vi "AlliGator Draw Phasor Plot SEPL v2.vi"(7 "Font, Size & Style":T1, 8 "Error In":errorcluster, 9 "Overlay Group":string="SEPL", 10 "Phasor Plot Reference Points":T2, 11 "Phasor Plot Image  in":T3) -> (0 "Error Out":errorcluster, 3 "Phasor Plot Image out":T3)   [LabVIEW 2021, in "AlliGator Phasor Plot.lvlib"]
doc: "Draws the selected SEPL on the Phasor Plot image."
uses:
  AlliGator Phasor Plot.lvlib
  <vilib>/vision/Image Controls.llb/IMAQ Image.ctl
  Phasor Ratio/AlliGator Phasor Plot Reference Points.ctl
  Settings/AlliGator Phasor Plot Graphics Options.ctl
  Settings/AlliGator Settings List.ctl
  92607714-a441-4b97-ba68-5943c871a3f7.vi
  Phasor Graph/AlliGator Phasor Graph.lvlib
  Settings/AlliGator Settings.lvlib
  Phasor Ratio/AlliGator Phasor Ratio.lvlib
panel:
  # "see the AlliGator License on the block diagram (Ctrl+E or Window:Show Block Diagram)"
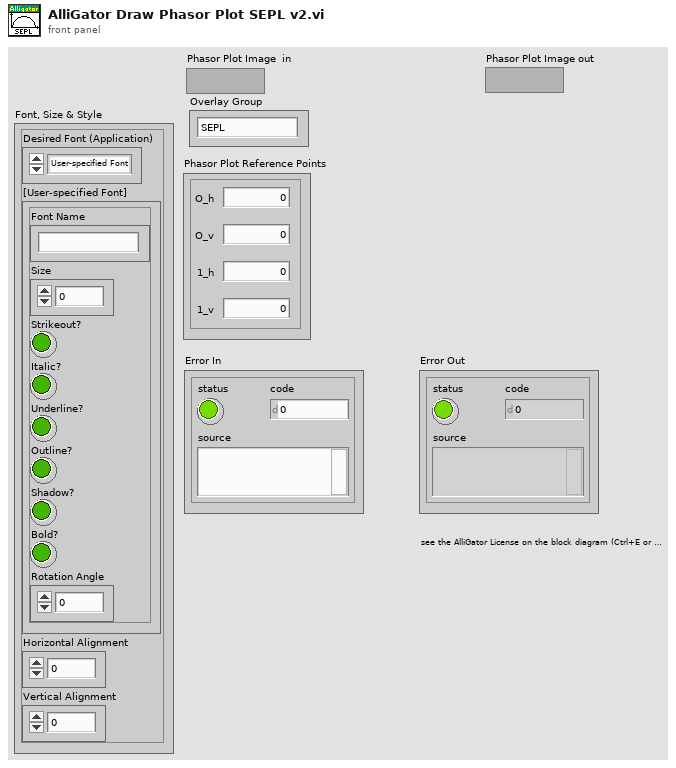
[diagram p1: front panel]
types:
  T1 = cluster{"Desired Font (Application)":enum16{"User-specified Font", "Application Font", "System Font", "Dialog Font"}, "[User-specified Font]":cluster{"Font Name":string, "Size":i16, "Strikeout?":bool, "Italic?":bool, "Underline?":bool, "Outline?":bool, "Shadow?":bool, "Bold?":bool, "Rotation Angle":dbl}, "Horizontal Alignment":i16, "Vertical Alignment":i16}
  T2 = typedef "AlliGator Phasor Ratio.lvlib/AlliGator Phasor Plot Reference Points.ctl" = cluster{"O_h":dbl, "O_v":dbl, "1_h":dbl, "1_v":dbl}
  T3 = typedef "IMAQ Image.ctl" = refnum<image>
  T4 = typedef "AlliGator Settings.lvlib/AlliGator Phasor Plot Graphics Options.ctl" = cluster{"UC Color":u32, "Show UC Tau Ticks":bool, "SEPL Color":u32, "Show SEPL Tau Ticks":bool, "Axes Color":u32, "Show (g,s) Ticks":bool, "Show UC":bool, "Show SEPL":bool, "Show Axes":bool, "Show UC Tau Labels":bool, "Show SEPL Tau Labels":bool, "Show (g,s) Labels":bool, "UC Label Size":i16, "UC Label Distance":dbl, "SEPL Label Size":i16, "SEPL Label Distance":dbl, "Axes Label Size":i16, "Axes Label Distance":dbl}
  T5 = typedef "AlliGator Settings.lvlib/AlliGator Settings List.ctl" = enum16{"GUI:Visible Settings Tab", "GUI:Last Run Version", "Source Image:Use Image Histogram for Contrast", "Source Image:Low Count Pixels Rejection Options", "Source Image:High Count Pixels Rejection Options", "Source Image:Use Image Brightness", "Source Image:Blend Overlay with Image Background", "Source Image:Use Fixed ROI Diameter", "Source Image:ROI Diameter", "Source Image:ROI Center Color", "Source Image:Peak Threshold", "Source Image:Intensity Threshold", "Source Image:Image Binning Options", "Source Image:Image Smoothing Options", "Source Image:Image Histogram Active", "Source Image:Invert Binary Mask", "Source Image:Hot Pixel Removal", "Source Image:Overlay Analyzed ROI Center", "Source Image:Auto-Adjust Contrast", "Source Image:Histogram Lower Percentile", "Source Image:Histogram Upper Percentile", "Source Image:Save Source Image", "Source Image:Scale Bar Options", "Source Image:Image Resolution (Pixel Size)", "Source Image:Flatfield Correction", "Source Image:Show Dead Left Columns Correction", "Source Image:Dead Left Columns Correction", "Source Image:Image Pre-Processing Operations Order", "Source Image:Overlay ROI Median", "Source Image:Median Overlay Color", "Data Information:Gate Width", "Data Information:Nanotime Gate Separation", "Data Information:Macrotime Gate Separation", "Data Information:Gate Step", "Data Information:# Gates", "Data Information:Gate Image Exposure", "Data Information:Gate Image Integration", "Data Information:Gates to Skip", "Data Information:Gates to Keep", "Data Information:Define Gates to", "Data Information:Channel Name", "Data Information:Available Channel Names", "Data Information:Channel Arithmetic", "Data Information:Background File Subtraction", "Data Information:Background File", "Data Information:Background Scaling Factor", "Data Information:Background Pile-up Correction", "Data Information:Background Pixel Well Capacity", "Data Information:Laser Period", "Data Information:SYNC Period", "Data Information:Pile-up Correction", "Data Information:Pixel Well Capacity", "Data Information:Dataset Scaling Factor", "Fluorescence Decay_Decay Pre-Processing:Reverse Gates", "Fluorescence Decay_Decay Pre-Processing:Verbose Decay Pre-Processing", "Fluorescence Decay_Decay Pre-Processing:Use Decay Pre-Processing", "Fluorescence Decay_Decay Pre-Processing:Background Subtraction", "Fluorescence Decay_Decay Pre-Processing:Background Definition Range", "Fluorescence Decay_Decay Pre-Processing:Baseline Subtraction Method", "Fluorescence Decay_Decay Pre-Processing:Decay Pre-Processing Operations Order", "Fluorescence Decay_Decay Pre-Processing:Smoothing Parameter", "Fluorescence Decay_Decay Pre-Processing:Shift Decay", "Fluorescence Decay_Decay Pre-Processing:Decay Shift Parameters", "Fluorescence Decay_Decay Pre-Processing:Fold Decay", "Fluorescence Decay_Decay Pre-Processing:# Folds", "Fluorescence Decay_Decay Pre-Processing:1-Normalize Decay", "Fluorescence Decay_Decay Pre-Processing:[0-1]-Normalize Decay", "Fluorescence Decay_Decay Pre-Processing:Smoothen Decay", "Fluorescence Decay_Decay Pre-Processing:Extrapolate Decay", "Fluorescence Decay_Decay Pre-Processing:Use Periodicity", "Fluorescence Decay_Decay Pre-Processing:Use Cursors", "Fluorescence Decay_Decay Pre-Processing:Tail Fraction", "Fluorescence Decay_Decay Pre-Processing:Head Fraction", "Fluorescence Decay_Decay Pre-Processing:Additional Points", "Fluorescence Decay_Decay Pre-Processing:Straighten Decay", "Fluorescence Decay_Decay Pre-Processing:Constant Background", "Fluorescence Decay_Decay Pre-Processing:Pixel-Normalize Decay", "Fluorescence Decay_Advanced Analysis:Extract IRF instead of Decay", "Fluorescence Decay_Advanced Analysis:IRF Extraction Options", "Fluorescence Decay_Advanced Analysis:IRF Optimization Options", "Fluorescence Decay_Advanced Analysis:Square Pulse Options", "Fluorescence Decay_Advanced Analysis:IRF Order", "Fluorescence Decay_Advanced Analysis:IRF Time Constants", "Fluorescence Decay_Advanced Analysis:Wavelet Analysis Options", "Fluorescence Decay_Advanced Analysis:Average Lifetime Options", "Fluorescence Decay_Fit Options:Fit Options", "Fluorescence Decay_Fit Options:Use Legacy Fitting Approach", "Fluorescence Decay_Fit Options:Use Data Information Laser Period", "Fluorescence Decay_Fit Parameters:Displayed Fit Parameters", "Fluorescence Decay_Fit Parameters:Fit Parameter Constraints", "Fluorescence Decay_Fit Parameters:Export Tabulated Results", "Fluorescence Decay_Fit Parameters:MLE Baseline Offset Type", "Fluorescence Decay_Fit Parameters:MLE Baseline Offset", "Fluorescence Decay_Fit Parameters:Guess Parameter Names", "Fluorescence Decay_Fit Parameters:Guess Parameter Values", "Fluorescence Decay_Fit Parameters:Guess Parameters Options", "Fluorescence Decay_Styles:Show Last Decay Only", "Fluorescence Decay_Styles:Decay Graph Color Array", "Fluorescence Decay:Decay Graph Active", "Fluorescence Decay Statistics:Min Peak Value", "Fluorescence Decay Statistics:Reject Low Decay Peak Pixels", "Fluorescence Decay Statistics:Reject High Decay Peak Pixels", "Fluorescence Decay Statistics:Max Peak Value", "Time Traces:Use File Timestamp", "Time Traces:Time Step", "Time Traces:Use Intensity Correction File", "Time Traces:Intensity Correction File", "Phasor Plot:Phasor Plot Smoothing Options", "Phasor Plot:Phasor Plot Size", "Phasor Plot:Phasor Plot Graphics Options", "Phasor Plot:Cumulative Phasor Plot", "Phasor Plot:Use Phasor Brightness", "Phasor Plot:Blend Overlay with Phasor Background", "Phasor Plot:Save Phasor Plot", "Phasor Plot:Show References", "Phasor Plot:Phasor Ratio Decay Range", "Phasor Plot:Exponential Fading", "Phasor Plot:Phasor Ratio Reference Colors", "Phasor Plot:Reference Radius", "Phasor Plot:Show Color Map Vertices", "Phasor Plot:Phasor Plot Active", "Phasor Plot:Phasor Ratio Color Map Type", "Phasor Plot:Phasor Ratio Color Map", "Phasor Plot:Phasor Ratio Display Range", "Phasor Plot:Selected Image ROI(s)", "Phasor Plot:All Image ROIs", "Phasor Plot:Selected Phasor Plot ROI(s)", "Phasor Plot:All Phasor Plot ROIs", "Phasor Plot:Phasor Ratio Color-Coded Quantity", "Phasor Plot:Store Phasor Harmonics", "Phasor Plot:Draw Reference Segment", "Phasor Plot:User-Defined Quantity", "Phasor Graph:Phasor Frequency", "Phasor Graph:Phasor Ratio Type", "Phasor Graph:Pixel-level Phasor Computation", "Phasor Graph:Save Phasor Graph", "Phasor Graph:Phasor Graph Active", "Phasor Graph:Phasor SDV Options", "Phasor Calibration:Use Backup Calibration if needed", "Phasor Graph:Define Shortest Lifetime as", "Phasor Calibration:Backup Calibration Type", "Phasor Calibration:Calibration Type", "Phasor Calibration:Calibration Lifetime", "Phasor Calibration:Calibration Map Algorithm", "Single-Exponential Phasor Locus (SEPL):Gate Parameters", "Single-Exponential Phasor Locus (SEPL):User-defined Gate", "Single-Exponential Phasor Locus (SEPL):User-defined IRF", "Single-Exponential Phasor Locus (SEPL):Phasor Parameters", "Single-Exponential Phasor Locus (SEPL):Decay & IRF Parameters", "Single-Exponential Phasor Locus (SEPL):Display Parameters", "Lifetime Analysis:Decay Analysis Parameters", "Lifetime Analysis:Lifetime Map Active", "Plugins:Python Settings", "Miscellaneous:Verbose Mode", "Miscellaneous:Beep after Script", "Miscellaneous:Saved Image File Format", "Miscellaneous:Exported Gate Image Settings", "Miscellaneous:Include Loading in Timing", "Miscellaneous:Verbose Settings Mode", "Miscellaneous:Histogram Options", "Miscellaneous:Beep on Error", "Miscellaneous:# Logical Processors Used", "Miscellaneous:ROI Description Max Characters", "Miscellaneous:Verbose Error Mode", "Miscellaneous:Transparent Mask Color"}
  T6 = typedef "Phasor.lvlib/Phasor SEPL Tick Data.ctl" = cluster{"tau_i (ns)":dbl, "Tick start (g, s)":T7, "Tick (dg, ds)":T7, "long tick?":bool}
  T7 = typedef "Phasor.lvlib/Phasor (g, s).ctl" = cluster{"g":dbl, "s":dbl}
  T8 = cluster{"Phasor Plot x":i32, "Phasor Plot y":i32}[]
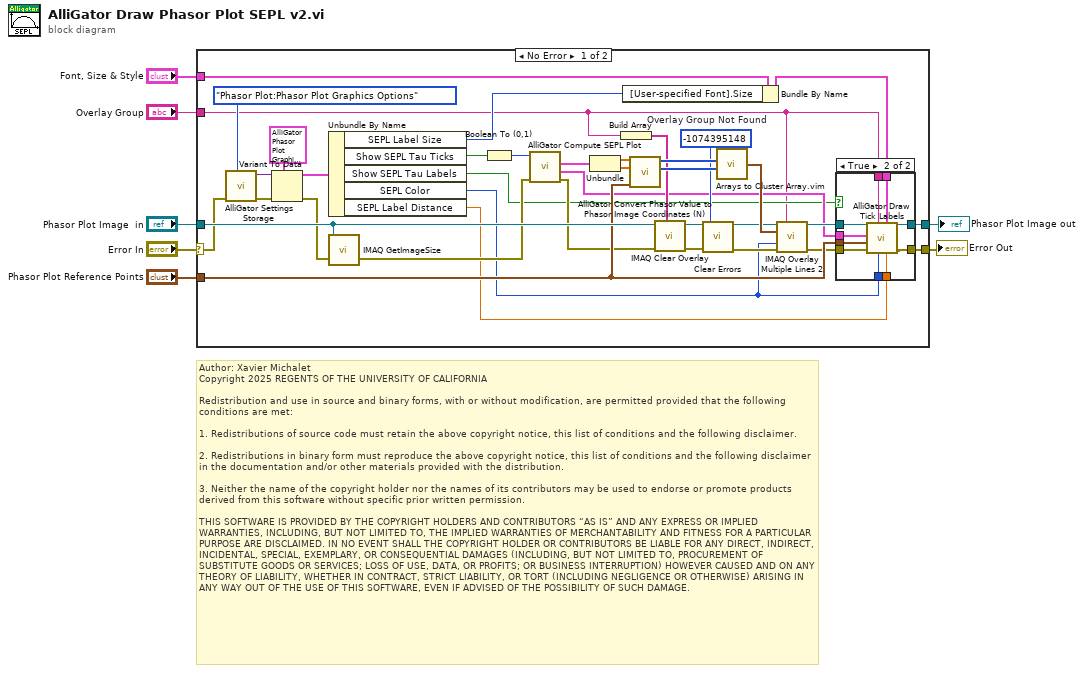
[diagram p0: block diagram]
diagram:
  # "Author: Xavier Michalet\nCopyright 2025 REGENTS OF THE UNIVERSITY OF CALIFORNIA\n\nRedistribution and use in source and binary forms, with or without modification, are permitted provided that the following conditions are met:\n\n1. Redistributions of source code must retain the above copyright notice, this list of conditions and the following disclaimer.\n\n2. Redistributions in binary form must reproduce the above copyright notice, this list of conditions and the following disclaimer in the documentation and/or other materials provided with the distribution.\n\n3. Neither the name of the copyright holder nor the names of its contributors may be used to endorse or promote products derived from this software without specific prior written permission.\n\nTHIS SOFTWARE IS PROVIDED BY THE COPYRIGHT HOLDERS AND CONTRIBUTORS “AS IS” AND ANY EXPRESS OR IMPLIED WARRANTIES, INCLUDING, BUT NOT LIMITED TO, THE IMPLIED WARRANTIES OF MERCHANTABILITY AND FITNESS FOR A PARTICULAR PURPOSE ARE DISCLAIMED. IN NO EVENT SHALL THE COPYRIGHT HOLDER OR CONTRIBUTORS BE LIABLE FOR ANY DIRECT, INDIRECT, INCIDENTAL, SPECIAL, EXEMPLARY, OR CONSEQUENTIAL DAMAGES (INCLUDING, BUT NOT LIMITED TO, PROCUREMENT OF SUBSTITUTE GOODS OR SERVICES; LOSS OF USE, DATA, OR PROFITS; OR BUSINESS INTERRUPTION) HOWEVER CAUSED AND ON ANY THEORY OF LIABILITY, WHETHER IN CONTRACT, STRICT LIABILITY, OR TORT (INCLUDING NEGLIGENCE OR OTHERWISE) ARISING IN ANY WAY OUT OF THE USE OF THIS SOFTWARE, EVEN IF ADVISED OF THE POSSIBILITY OF SUCH DAMAGE."
  n1 = case shown="No Error" "Error In" {
    selector: "Error In" -> [w19 w56]
    tunnel: [w43 w57] -> w7
    tunnel: [w42 w56] -> w6
    tunnel: "Phasor Plot Image  in" -> [w41 w57]
    tunnel: "Phasor Plot Reference Points" -> [w40 _]
    tunnel: "Font, Size & Style" -> [w39 _]
    tunnel: "Overlay Group" -> [w8 _]
    frame No Error {
      w29 = -1074395148  # Overlay Group Not Found
      n2 = call "AlliGator Settings Storage.vi"("AlliGator Settings List"=AlliGator_Settings_List."Phasor Plot:Phasor Plot Graphics Options", "Error In"=w19) -> ("Error Out"=w20:errorcluster, "Variant Data out"=w21:variant)  [unwired: 8 in]
      n3 = Variant To Data(error in=w20, type=T4 {"UC Color"=3381759, "Show UC Tau Ticks"=FALSE, "SEPL Color"=3381759, "Show SEPL Tau Ticks"=FALSE, "Axes Color"=16776960, "Show (g,s) Ticks"=FALSE, "Show UC"=FALSE, "Show SEPL"=FALSE, "Show Axes"=FALSE, "Show UC Tau Labels"=FALSE, "Show SEPL Tau Labels"=FALSE, "Show (g,s) Labels"=FALSE, "UC Label Size"=18, "UC Label Distance"=0.0, "SEPL Label Size"=18, "SEPL Label Distance"=0.0, "Axes Label Size"=18, "Axes Label Distance"=0.0} ("Phasor Plot Graphics Options"), Variant=w21) -> (data=w16:T4, error out=w18:errorcluster)
      n4 = Unbundle By Name(w16) -> ("SEPL Label Size"=w9:i16, "Show SEPL Tau Ticks"=w15:bool, "Show SEPL Tau Labels"=w14:bool, "SEPL Color"=w13:u32, "SEPL Label Distance"=w11:dbl)
      n5 = call "IMAQ GetImageSize"("Image"=w41, "error in (no error)"=w18) -> ("error out"=w28:errorcluster)  [unwired: 2 in, 2 out]
      n6 = Boolean To (0,1)(Boolean=w15) -> (0, 1=w12:i16)
      n7 = call "AlliGator Compute SEPL Plot.vi"("Error In"=w28, "Show Ticks? (Use SEPL Settings)"=w12) -> ("error out"=w27:errorcluster, "Tick Label Data"=w23:T6[], "SEPL Plot"=w26:cluster{"X Array":dbl[], "Y Array":dbl[]})  [unwired: 6 in, 1 out]
      n8 = Unbundle(w26) -> ("X Array"=w38:dbl[], "Y Array"=w37:dbl[])
      n9 = Build Array(w8) -> (w33:string[])
      n10 = Bundle By Name(cluster=w39, "[User-specified Font].Size"=w9) -> (w10:T1)
      n11 = call "AlliGator Convert Phasor Value to Phasor Image Coordinates (N).vi"("Phasor Plot Reference Points"=w40, "Phasor s"=w37, "Phasor g"=w38) -> ("Phasor Plot y"=w35:i32[], "Phasor Plot x"=w36:i32[])  [unwired: 7 in]
      n12 = call "IMAQ Clear Overlay"("Groups"=w33, "error in (no error)"=w27, "Image"=w41) -> ("error out"=w32:errorcluster, "Image Out"=w30:T3)  [unwired: 7 in]
      n13 = call <vilib>:"Clear Errors.vi"("error in (no error)"=w32, "specific error code to clear (0: all)"=w29) -> ("error out"=w31:errorcluster)  [unwired: 4 in, 1 out]
      n14 = call "Arrays to Cluster Array.vim"("Array 1"=w36, "Array 2"=w35) -> ("Cluster Array"=w34:T8)  [unwired: 6 in]
      n15 = call "IMAQ Overlay Multiple Lines 2"("Image"=w30, "Group"=w8, "Line End Points"=w34, "Color"=w13, "error in (no error)"=w31) -> ("Image Out"=w25:T3, "error out"=w24:errorcluster)  [unwired: 9 in]
      n16 = case shown="True" w14 {
        tunnel: [w45 w55] -> w43
        tunnel: [w44 w54] -> w42
        tunnel: w13 -> [_ w53]
        tunnel: w40 -> [_ w52]
        tunnel: w10 -> [_ w51]
        tunnel: w25 -> [w45 w50]
        tunnel: w24 -> [w44 w49]
        tunnel: w8 -> [_ w48]
        tunnel: w23 -> [_ w47]
        tunnel: w11 -> [_ w46]
        frame False {
        }
        frame True {
          n17 = call "AlliGator Draw Tick Labels.vi"("Label Distance (tick unit)"=w46, "Font, Size & Style"=w51, "Text Color"=w53, "Overlay Group"=w48, "error in (no error)"=w49, "Phasor Plot Reference Points"=w52, "Tick Label Data"=w47, "Refnum in"=w50) -> ("error out"=w54:errorcluster, "Refnum out"=w55:T3)  [unwired: 2 in]
        }
      }
    }
    frame Error {
    }
  }
  "Phasor Plot Image out" <- w7
  "Error Out" <- w6
